vi "SetScale.vi"(6 "Axis":enum16{"x", "y", "z"}(ring), 8 "error in (no error)":errorcluster, 9 "wavename (Axis)":string, 10 "wavename (Image)":string, 11 "ITX Commands in":refnum<class "ITX Commands.lvclass">) -> (0 "error out":errorcluster, 3 "ITX Commands out":refnum<class "ITX Commands.lvclass">)   [LabVIEW 2019, in "ITX Commands.lvclass"]
uses:
  ITX Commands.lvclass
  ITX Commands.lvclass/ITX Commands.ctl
panel:
  out "Command String":string
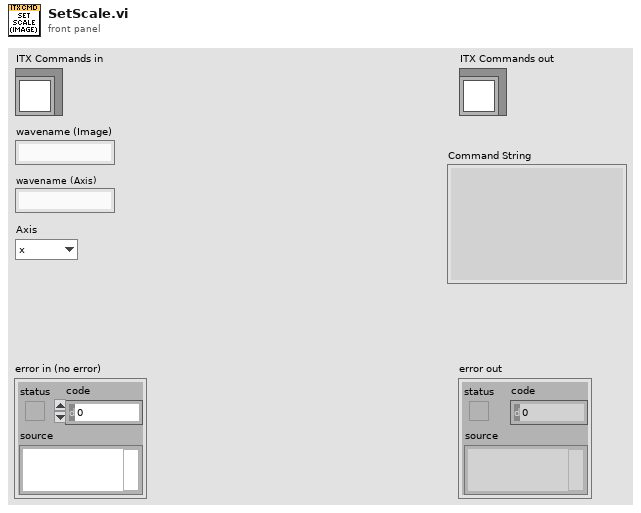
[diagram p1: front panel]
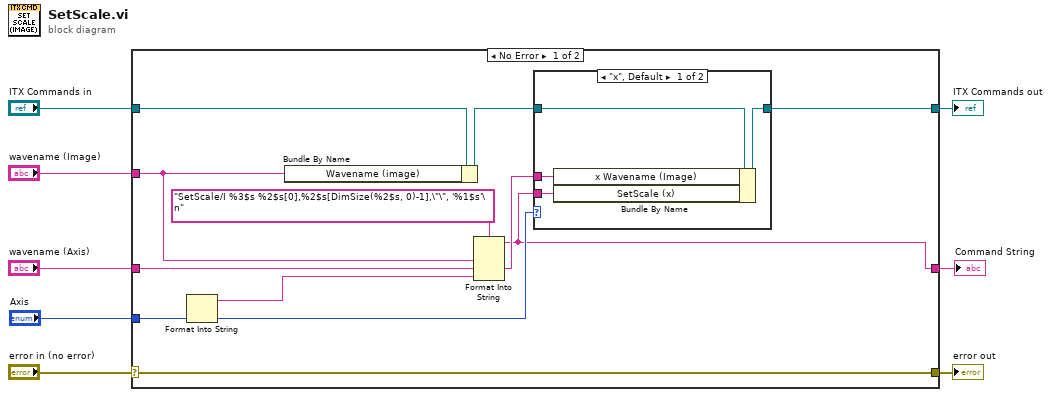
[diagram p0: block diagram]
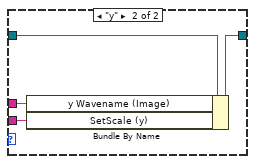
[diagram p2: hidden frame]
diagram:
  n1 = case shown="No Error" "error in (no error)" {
    selector: "error in (no error)" -> [w16 w28]
    tunnel: [w16 w28] -> w7
    tunnel: [w10 w27] -> w5
    tunnel: "ITX Commands in" -> [w18 w27]
    tunnel: "wavename (Image)" -> [w15 _]
    tunnel: "wavename (Axis)" -> [w11 _]
    tunnel: [w9 _] -> w3
    tunnel: "Axis" -> [w13 _]
    frame No Error {
      n2 = Format Into String(w13) -> (resulting string=w14:string)  [unwired: 3 in, 1 out]
      n3 = Bundle By Name(cluster=w18, "Wavename (image)"=w15) -> (w12:refnum<class "ITX Commands.lvclass">)
      n4 = Format Into String(format string="SetScale/I %3$s %2$s[0],%2$s[DimSize(%2$s, 0)-1],\"\", '%1$s'\n" ("input string 1"), w15, w11, w14) -> (resulting string=w9:string)  [unwired: 2 in, 1 out]
      n5 = case shown="\"x\", Default" w13 {
        tunnel: w12 -> [w21 w26]
        tunnel: w11 -> [w22 w25]
        tunnel: [w20 w24] -> w10
        tunnel: w9 -> [w19 w23]
        frame "x", Default {
          n6 = Bundle By Name(cluster=w21, "x Wavename (Image)"=w22, "SetScale (x)"=w19) -> (w20:refnum<class "ITX Commands.lvclass">)
        }
        frame "y" {
          n7 = Bundle By Name(cluster=w26, "y Wavename (Image)"=w25, "SetScale (y)"=w23) -> (w24:refnum<class "ITX Commands.lvclass">)
        }
      }
    }
    frame Error {
    }
  }
  "error out" <- w7
  "ITX Commands out" <- w5
  "Command String" <- w3
